vi "Test Dynamic Load Classes.vi"() -> ()   [LabVIEW 2019, in "Control Experiment.lvclass"]
uses:
  Control Experiment.lvclass
  <userlib>/LevyLab/Instrument Framework/Instrument Types/Amplifier/Instrument.Amplifier.lvclass
  <userlib>/LevyLab/Krohn Hite 7008/Inst.Krohn-Hite-7008/Inst.Krohn-Hite-7008.lvclass
  Control Experiment.lvclass/Control Experiment.ctl
panel:
  out "specific class reference":refnum<class "Inst.Krohn-Hite-7008.lvclass">
  out "Instrument Classes.KH7008":refnum<class "Instrument.Amplifier.lvclass">
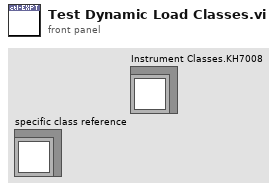
[diagram p1: front panel]
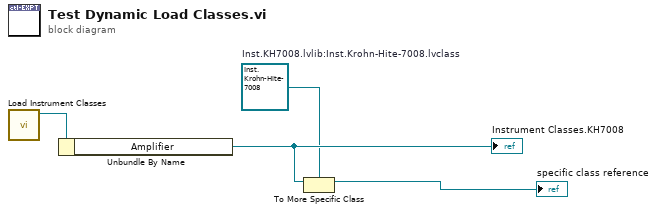
[diagram p0: block diagram]
diagram:
  w2 = refnum<class "Inst.Krohn-Hite-7008.lvclass"> refnum  # Inst.KH7008.lvlib:Inst.Krohn-Hite-7008.lvclass
  n1 = call "Load Instrument Classes.vi"() -> ("Control Experiment"=w4:refnum<class "Control Experiment.lvclass">)  [unwired: 10 in, 1 out]
  n2 = Unbundle By Name(w4) -> ("Amplifier"=w3:refnum<class "Instrument.Amplifier.lvclass">)
  "Instrument Classes.KH7008" <- w3
  n3 = To More Specific Class(target class=w2, reference=w3) -> (specific class reference=→"specific class reference":refnum<class "Inst.Krohn-Hite-7008.lvclass">)  [unwired: 1 in, 1 out]
